vi "RMPS Globals.vi"() -> ()   [LabVIEW 2025]
doc: "Author: Scott Hannahs <sth@magnet.fsu.edu>\n\nThis software is licensed for use under the “MIT License\"\nCopyright (c) 2025 Scott Hannahs, sth@sth@magnet.sthnet.net\n\nPermission is hereby granted, free of charge, to any person obtaining a copy of this software and associated documentation files (the \"Software\"), to deal in the Software without restriction, including without limitation the rights to use, copy, modify, merge, publish, distribute, sublicense, and/or sell copies of the Software, and to permit persons to whom the Software is furnished to do so, subject to the following conditions: The above copyright notice and this permission notice shall be included in all copies or substantial portions of the Software.\n\nTHE SOFTWARE IS PROVIDED \"AS IS\", WITHOUT WARRANTY OF ANY KIND, EXPRESS OR IMPLIED, INCLUDING BUT NOT LIMITED TO THE WARRANTIES OF MERCHANTABILITY, FITNESS FOR A PARTICULAR PURPOSE AND NONINFRINGEMENT. IN NO EVENT SHALL THE AUTHORS OR COPYRIGHT HOLDERS BE LIABLE FOR ANY CLAIM, DAMAGES OR OTHER LIABILITY, WHETHER IN AN ACTION OF CONTRACT, TORT OR OTHERWISE, ARISING FROM, OUT OF OR IN CONNECTION WITH THE SOFTWARE OR THE USE OR OTHER DEALINGS IN THE SOFTWARE."
panel:
  in  "# Cycles To Activate":u32=5
  in  "Actual Cycle Time":dbl format="%.6f"
  in  "Recording Interval":dbl=2.0 format="%.1f"
  out "RMPS Data Queue":refnum<queue>
  in  "Activation Current":dbl=1.0 format="%.1f"
  in  "# Non-coil Channels":u32=11
  in  "Max Board Acq Rate":dbl=95000.0
  in  "Cycle Freq":dbl=30.0 format="%.3f"
  out "DAQ Buffer Size":u32
  in  "Posttrigger Sec of Data":dbl=10.0 format="%.2f"
  in  "Pretrigger sec of data":dbl=30.0 format="%.2f"
  in  "Magnet Data":dbl[](array[numeric]) format="%.3f"
  in  "# Scans to read":i32
  out "Seconds/Scan":dbl format="%^.4e"
  out "Digital  IO Task":refnum<k21>
  out "Analog taskID":refnum<k21>
  out "# Coils":u32
  # "Tin"
  # "Tout"
  # "Pin"
  # "Pout"
  # "Current"
  # "WDTimer"
  # "PSenb"
  # "Cell Fault"
  # "WDTrip"
  # "BT Trip"
  # "BT Volts"
  # "Va"
  # "Vb"
  # "Vc"
  # "Vd"
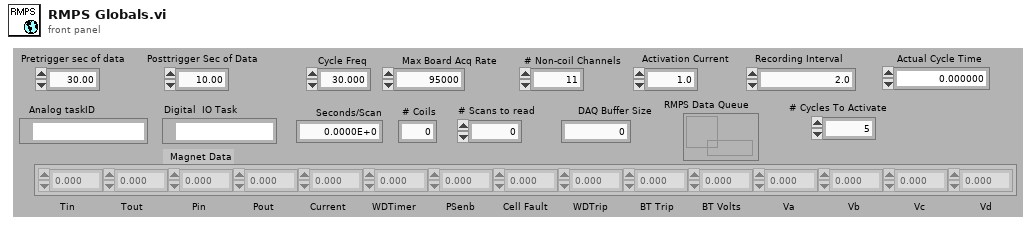
[diagram p1: front panel]
diagram:
